vi "Identities.vi"(8 "error in (no error)":errorcluster, 11 "ConfigAPI in":refnum<class "ConfigAPI.lvclass">) -> (0 "error out":errorcluster, 2 "Identities":refnum<class "Identity.lvclass">[](array[class]), 3 "ConfigAPI out":refnum<class "ConfigAPI.lvclass">)   [LabVIEW 2020, in "Volatus.lvlib" / "ConfigAPI.lvclass"]
uses:
  ConfigAPI.lvclass
  Identity/Identity.lvclass
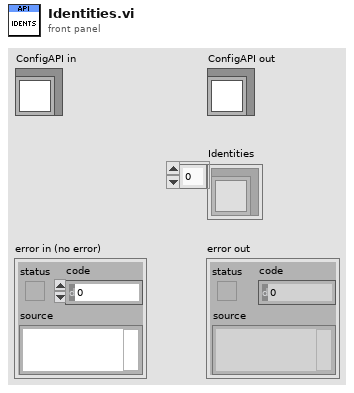
[diagram p1: front panel]
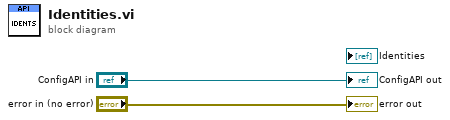
[diagram p0: block diagram]
diagram:
  "error out" <- "error in (no error)"
  "ConfigAPI out" <- "ConfigAPI in"
